vi "Write Serial data.vi"(8 "error in":errorcluster, 10 "PAS Data In":refnum<class "PAS Data.lvclass">, 11 "File Obs in":refnum<class "PAS File Obs.lvclass">) -> (0 "error out":errorcluster, 2 "PAS Data Out":refnum<class "PAS Data.lvclass">, 3 "File Obs Out":refnum<class "PAS File Obs.lvclass">)   [LabVIEW 2015, in "PAS File Obs.lvclass"]
uses:
  PAS File Obs.lvclass
  Data/Main/PAS Data.lvclass
  Devices/Alicat/Session Based/Data/Alicat Data.lvclass
  Instruments/AOP/Data/cPAS Data.lvclass
  Devices/TE Cooler/Data/TECData.lvclass
  File IO/Class/File Observer.lvclass/File Observer.ctl
  Instruments/AOP/Data/cPAS Data.lvclass/cPAS Data.ctl
  Main/Controls/Cell Data.ctl
  Main/Controls/pas_data_enum.ctl
  File IO/Class/Read File Ref.vi
  Instruments/AOP/Data/Read Serial Data.vi
  Data/Data.lvclass
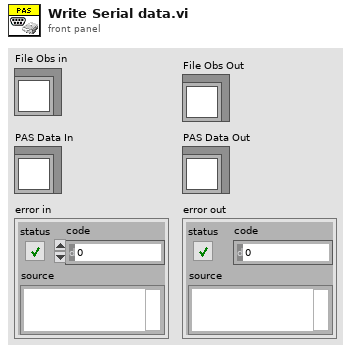
[diagram p1: front panel]
types:
  T1 = enum16{"big-endian, network order", "native, host order", "little-endian"}
  T2 = typedef "Cell Data.ctl" = u8
  T3 = typedef "pas_data_enum.ctl" = enum8{"Time", "Ttec", "tecPow", "Spk Position", "Spk Amplification", "Vspan", "Modulation", "Vspk", "Filter", "DC State", "Notes", "O3 Flag", "Raw Flags"}
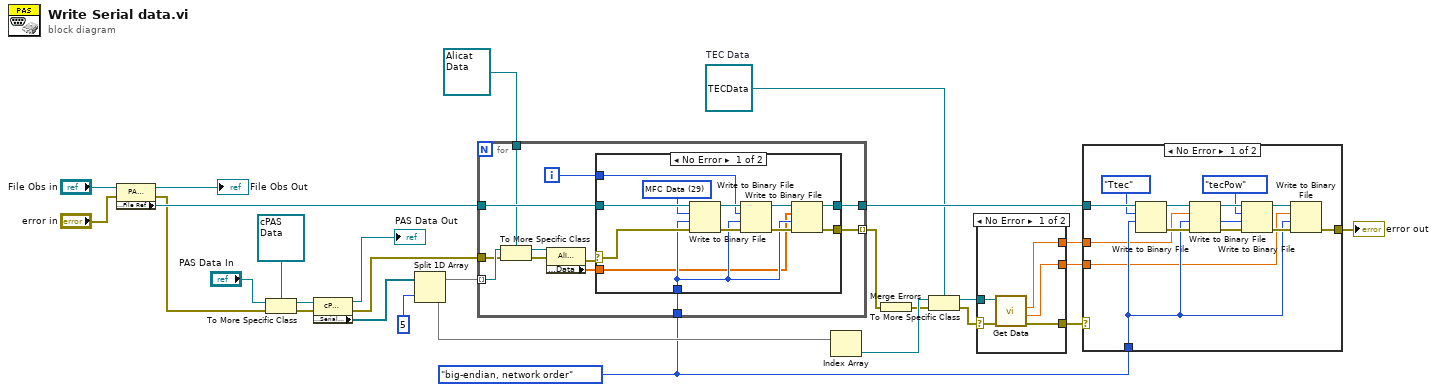
[diagram p0: block diagram]
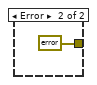
[diagram p3: hidden frame]
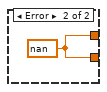
[diagram p4: hidden frame]
diagram:
  w1 = refnum<class "TECData.lvclass"> refnum  # TEC Data
  w15 = T1."big-endian, network order" ("byte order (0:big-endian, network order)")
  n1 = property class="PAS File Obs"(reference="File Obs in", error in="error in") -> (reference out=→"File Obs Out":refnum<class "PAS File Obs.lvclass">, error out=w6:errorcluster, "Data Access:File Ref"=w16:refnum<file>)
  n2 = To More Specific Class(target class=refnum<class "cPAS Data.lvclass"> refnum ("cPAS Data"), reference="PAS Data In", error in=w6) -> (specific class reference=w7:refnum<class "cPAS Data.lvclass">, error out=w5:errorcluster)
  n3 = property class="cPAS Data"(reference=w7, error in=w5) -> (reference out=→"PAS Data Out":refnum<class "cPAS Data.lvclass">, error out=w3:errorcluster, "Accessors:Serial Data"=w4:refnum<class "Data.lvclass">[])
  n4 = Split 1D Array(array=w4, index=5) -> (first subarray=w17:refnum<class "Data.lvclass">[], second subarray=w26:refnum<class "Data.lvclass">[])
  n5 = for {
    tunnel: w17 -> [w40] mode=indexing
    tunnel: w16 -> [w39]
    tunnel: [w38] -> w14
    tunnel: w3 -> [w37]
    tunnel: w15 -> [w36]
    tunnel: [w34] -> w13 mode=indexing
    tunnel: refnum<class "Alicat Data.lvclass"> refnum ("Alicat Data") -> [w33]
    i -> [w35]
    n6 = To More Specific Class(target class=w33, reference=w40, error in=w37) -> (specific class reference=w32:refnum<class "Alicat Data.lvclass">, error out=w31:errorcluster)
    n7 = property class="Alicat Data"(reference=w32, error in=w31) -> (error out=w29:errorcluster, "Accessors:Data"=w30:sgl[])  [unwired: 1 out]
    n8 = case shown="No Error" w29 {
      selector: w29 -> [w43 w53]
      tunnel: w39 -> [w52 w54]
      tunnel: [w47 w53] -> w34
      tunnel: [w45 w54] -> w38
      tunnel: w36 -> [w42 _]
      tunnel: w35 -> [w44 _]
      tunnel: w30 -> [w41 _]
      frame No Error {
        w46 = T2 29 items=["TEC SP"=23, "TEC Enable"=24, "MFC Data"=29, "Cell TEC T (T1)"=30, "Tmain"=31, "Tv"=32, "RHv"=33, "lasRMS"=34, "dPhi"=35, "Tau"=36, "Cell Q"=37, "f0"=38, "Integrated Area"=39, "Max Amplitude"=40, "Noise Limit"=41, "Lower Noise Bound"=42, "Upper Noise Bound"=43, "Absorption"=44, "fit params"=45, "covariance"=46] ("cellNumData")
        n9 = Write to Binary File(file (use dialog)=w52, data=w46, error in=w43, 9:w42) -> (refnum out=w51:refnum<file>, error out=w50:errorcluster)  [unwired: 2 in, 1 out]
        n10 = Write to Binary File(file (use dialog)=w51, data=w44, error in=w50, 9:w42) -> (refnum out=w49:refnum<file>, error out=w48:errorcluster)  [unwired: 2 in, 1 out]
        n11 = Write to Binary File(file (use dialog)=w49, data=w41, error in=w48, 9:w42) -> (refnum out=w45:refnum<file>, error out=w47:errorcluster)  [unwired: 2 in, 1 out]
      }
      frame Error {
      }
    }
  }
  n12 = Index Array(array=w26) -> (element=w20:refnum<class "Data.lvclass">)  [unwired: 1 in]
  n13 = Merge Errors(w13) -> (w12:errorcluster)
  n14 = To More Specific Class(target class=w1, reference=w20, error in=w12) -> (specific class reference=w22:refnum<class "TECData.lvclass">, error out=w24:errorcluster)
  n15 = case shown="No Error" w24 {
    selector: w24 -> [w56 _]
    tunnel: w22 -> [w59 _]
    tunnel: [w58 w60] -> w23
    tunnel: [w57 _] -> w28
    tunnel: [w55 w60] -> w27
    frame No Error {
      n16 = call "Get Data.vi"("error in (no error)"=w56, "TECData in"=w59) -> ("error out"=w57:errorcluster, "Power"=w55:sgl, "T"=w58:sgl)  [unwired: 6 in, 1 out]
    }
    frame Error {
      w60 = sgl nan ("T")
    }
  }
  n17 = case shown="No Error" w28 {
    tunnel: [w71 errorcluster {"status"=FALSE, "code"=0, "source"=""} ("error out")] -> w21
    tunnel: w23 -> [w62 _]
    tunnel: w15 -> [w65 _]
    tunnel: w27 -> [w61 _]
    tunnel: w14 -> [w66 _]
    frame No Error {
      n18 = Write to Binary File(file (use dialog)=w66, data=pas_data_enum."Ttec" ("Enum"), 9:w65) -> (refnum out=w70:refnum<file>, error out=w67:errorcluster)  [unwired: 3 in, 1 out]
      n19 = Write to Binary File(file (use dialog)=w70, data=w62, error in=w67, 9:w65) -> (refnum out=w69:refnum<file>, error out=w68:errorcluster)  [unwired: 2 in, 1 out]
      n20 = Write to Binary File(file (use dialog)=w69, data=pas_data_enum."tecPow" ("Enum"), error in=w68, 9:w65) -> (refnum out=w72:refnum<file>, error out=w73:errorcluster)  [unwired: 2 in, 1 out]
      n21 = Write to Binary File(file (use dialog)=w72, data=w61, error in=w73, 9:w65) -> (error out=w71:errorcluster)  [unwired: 2 in, 2 out]
    }
    frame Error {
    }
  }
  "error out" <- w21
